vi "MecaDriveKinematicsConstraint_getMinMaxAccel.vi"(8 "maxVelocity":dbl, 9 "Curvature":dbl, 10 "statePose":T6={"TRANSLATION"={"X"=0.0, "Y"=0.0}, "ROTATION"={"VALUE"=0.0, "COS"=1.0, "SIN"=0.0}} {"ROTATION"."SIN" format="%13.4f"; "ROTATION"."COS" format="%13.4f"; "ROTATION"."VALUE" format="%13.4f"; "TRANSLATION"."Y" format="%14.3f"; "TRANSLATION"."X" format="%14.3f"}, 11 "MECANUM_DRIVE_KINE_CONSTRAINT":T1={"Max Speed (M/S)"=0.0, "MECA_DRIVE_KINEMATICS"={"FrontLeft"={"X"=0.0, "Y"=0.0}, "FrontRight"={"X"=0.0, "Y"=0.0}, "RearLeft"={"X"=0.0, "Y"=0.0}, "RearRight"={"X"=0.0, "Y"=0.0}, "InverseKinematics"=[[0.0, 1.0, -1.0, 0.0], [0.0, 1.0, 1.0, 0.0], [0.0, 1.0, 1.0, 0.0], [0.0, 1.0, -1.0, 0.0]], "ForwardKinematics"=[[0.0, 1.0, -1.0, 0.0], [0.0, 1.0, 1.0, 0.0], [0.0, 1.0, 1.0, 0.0], [0.0, 1.0, -1.0, 0.0]], "PrevCoR"={"X"=0.0, "Y"=0.0}}} {"MECA_DRIVE_KINEMATICS"."PrevCoR"."Y" format="%14.3f"; "MECA_DRIVE_KINEMATICS"."PrevCoR"."X" format="%14.3f"; "MECA_DRIVE_KINEMATICS"."RearRight"."Y" format="%14.3f"; "MECA_DRIVE_KINEMATICS"."RearRight"."X" format="%14.3f"; "MECA_DRIVE_KINEMATICS"."RearLeft"."Y" format="%14.3f"; "MECA_DRIVE_KINEMATICS"."RearLeft"."X" format="%14.3f"; "MECA_DRIVE_KINEMATICS"."FrontRight"."Y" format="%14.3f"; "MECA_DRIVE_KINEMATICS"."FrontRight"."X" format="%14.3f"; "MECA_DRIVE_KINEMATICS"."FrontLeft"."Y" format="%14.3f"; "MECA_DRIVE_KINEMATICS"."FrontLeft"."X" format="%14.3f"; "Max Speed (M/S)" format="%20.4f"}) -> (3 "TRAJ_CONSTAINT_MIN_MAX":T5)   [LabVIEW 2019, in "Trajectory_Library.lvlib"]
doc: "Return the minimum and maximum allowed acceleration given the provided conditions.\n\nIt appears that this routine doesn't do anything. It returns default values.\n\nParameters:\n - MecanumDriveKinematicsConstraint - Constraint data structure\n - statePose - current traj state Pose\n - curvature - current traj curvature\n - maxVelocity - current traj max velocity\n\nReturns\n - TrajConstraint_Min_Max - Data structure with Min / Max acceleration."
uses:
  Trajectory_Library.lvlib
  POSE2D.ctl
  TRANSLATION2D.ctl
  ROTATION2D.ctl
  TRAJ_CONSTRAINT_MINMAX.ctl
  TRAJ_CONSTRAINT_MECA_DRIVE_KINEMATICS.ctl
  MECA_DRIVE_KINEMATICS.ctl
  <vilib>/Analysis/Matrix/Datatypes/RealMatrix.ctl
  <vilib>/Analysis/Matrix/NI_Matrix.lvlib
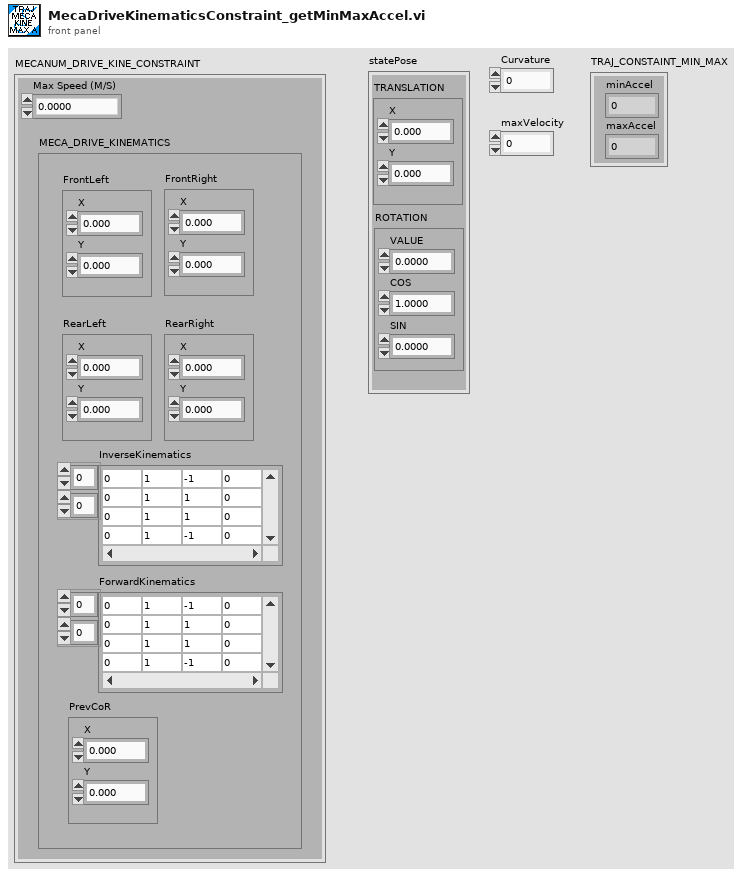
[diagram p1: front panel]
types:
  T1 = typedef "Trajectory_Library.lvlib/TRAJ_CONSTRAINT_MECA_DRIVE_KINEMATICS.ctl" = cluster{"Max Speed (M/S)":dbl, "MECA_DRIVE_KINEMATICS":T2}
  T2 = typedef "Trajectory_Library.lvlib/MECA_DRIVE_KINEMATICS.ctl" = cluster{"FrontLeft":T3, "FrontRight":T3, "RearLeft":T3, "RearRight":T3, "InverseKinematics":T4, "ForwardKinematics":T4, "PrevCoR":T3}
  T3 = typedef "Trajectory_Library.lvlib/TRANSLATION2D.ctl" = cluster{"X":dbl, "Y":dbl}
  T4 = typedef "NI_Matrix.lvlib/RealMatrix.ctl" = dbl[][]
  T5 = typedef "Trajectory_Library.lvlib/TRAJ_CONSTRAINT_MINMAX.ctl" = cluster{"minAccel":dbl, "maxAccel":dbl}
  T6 = typedef "Trajectory_Library.lvlib/POSE2D.ctl" = cluster{"TRANSLATION":T3, "ROTATION":T7}
  T7 = typedef "Trajectory_Library.lvlib/ROTATION2D.ctl" = cluster{"VALUE":dbl, "COS":dbl, "SIN":dbl}
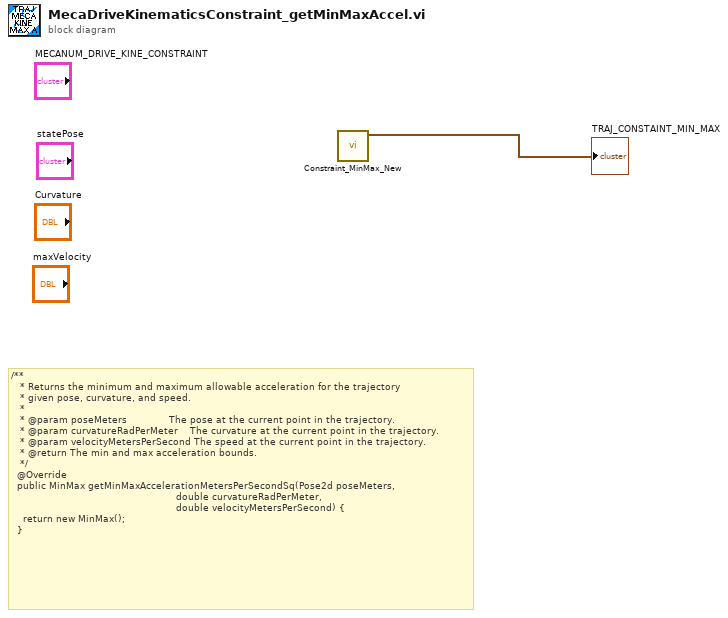
[diagram p0: block diagram]
diagram:
  # "/**\n   * Returns the minimum and maximum allowable acceleration for the trajectory\n   * given pose, curvature, and speed.\n   *\n   * @param poseMeters              The pose at the current point in the trajectory.\n   * @param curvatureRadPerMeter    The curvature at the current point in the trajectory.\n   * @param velocityMetersPerSecond The speed at the current point in the trajectory.\n   * @return The min and max acceleration bounds.\n   */\n  @Override\n  public MinMax getMinMaxAccelerationMetersPerSecondSq(Pose2d poseMeters,\n                                                       double curvatureRadPerMeter,\n                                                       double velocityMetersPerSecond) {\n    return new MinMax();\n  }"
  n1 = call "Constraint_MinMax_New.vi"() -> ("TRAJ_CONSTAINT_MIN_MAX"=→"TRAJ_CONSTAINT_MIN_MAX":T5)  [unwired: 11 in]
